vi "First Step.vi"(8 "error in (no error)":errorcluster, 11 "Wavelength PEM and Digikröm.lvclass in":refnum<class "Wavelength PEM and Digikröm.lvclass">) -> (0 "error out":errorcluster, 2 "Current Position":dbl, 3 "Wavelength PEM and Digikröm.lvclass out":refnum<class "Wavelength PEM and Digikröm.lvclass">)   [LabVIEW 2017, in "Wavelength PEM and Digikröm.lvclass"]
doc: "(Dynamic) Reset the instrument and prepare to scan. Go to step #0 - the first step. If desired, the scanner may do this in a different way than usual (i.e. by preparing to move a long distance, or reset to home position.)"
uses:
  Scanner/Scanner.lvclass
  Instruments/Utility Classes/Scannable/Scannable.lvclass
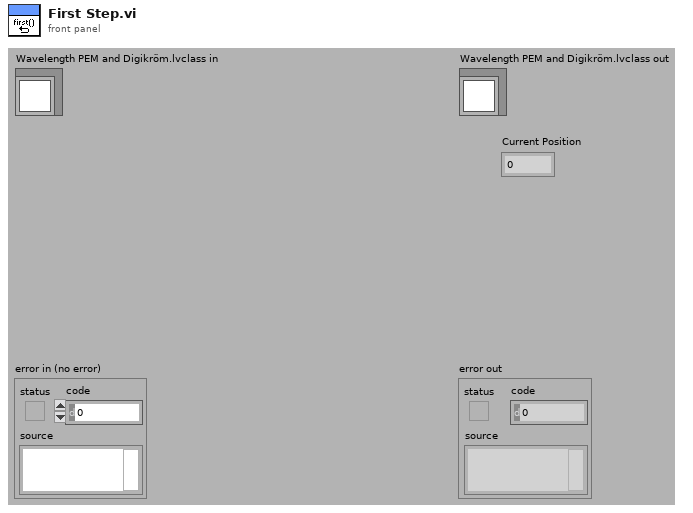
[diagram p1: front panel]
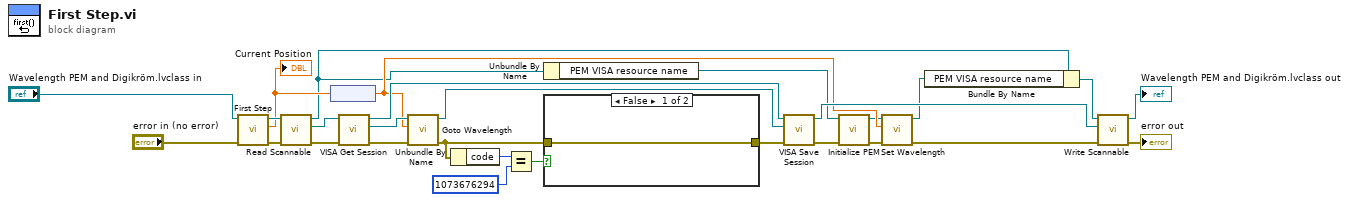
[diagram p0: block diagram]
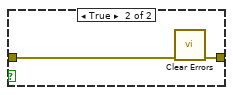
[diagram p2: hidden frame]
diagram:
  n1 = call-parent "First Step.vi"("error in (no error)"="error in (no error)", "Scanner.lvclass in"="Wavelength PEM and Digikröm.lvclass in") -> ("error out"=w20:errorcluster, "Current Position"=w13:dbl, "Scanner.lvclass out"=w24:refnum<class "Wavelength PEM and Digikröm.lvclass">)  [unwired: 7 out]
  "Current Position" <- w13
  n2 = call-dynamic "Read Scannable.vi"("error in (no error)"=w20, "Scanner.lvclass in"=w24) -> ("error out"=w19:errorcluster, "Scannable.lvclass"=w23:refnum<class "Scannable.lvclass">, "Scanner.lvclass out"=w8:refnum<class "Wavelength PEM and Digikröm.lvclass">)  [unwired: 7 out]
  n3 = node(w13) -> (w10:dbl[unit])
  n4 = call-dynamic "VISA Get Session.vi"("error in (no error)"=w19, "Instrument.lvclass in"=w23) -> ("error out"=w18:errorcluster, "VISA Resource Name"=w22:refnum<visa-resource-name>, "Instrument.lvclass out"=w16:refnum<class "Scannable.lvclass">)  [unwired: 7 out]
  n5 = call "Goto Wavelength.vi"("error in (no error)"=w18, "WAVELENGTH"=w10, "VISA resource name"=w22) -> ("error out"=w28:errorcluster, "VISA resource name out"=w21:refnum<visa-resource-name>)  [unwired: 7 out]
  n6 = Unbundle By Name(w28) -> ("code"=w26:i32)
  n7 = Equal?(x=w26, y=1073676294) -> (x = y?=w25:bool)
  n8 = Unbundle By Name(w8) -> ("PEM VISA resource name"=w1:refnum<visa-resource-name>)
  n9 = case shown="False" w25 {
    tunnel: w28 -> [w29 w31]
    tunnel: [w29 w30] -> w6
    frame False {
    }
    frame True {
      n10 = call <vilib>:"Clear Errors.vi"("error in (no error)"=w31) -> ("error out"=w30:errorcluster)  [unwired: 5 in, 1 out]
    }
  }
  n11 = call-dynamic "VISA Save Session.vi"("error in (no error)"=w6, "VISA Resource Name"=w21, "Instrument.lvclass in"=w16) -> ("error out"=w4:errorcluster, "Instrument.lvclass out"=w17:refnum<class "Scannable.lvclass">)  [unwired: 7 out]
  n12 = call "Initialize PEM.vi"("error in (no error)"=w4, "VISA resource name"=w1) -> ("error out"=w3:errorcluster, "VISA resource name out"=w2:refnum<visa-resource-name>)  [unwired: 8 in]
  n13 = call "Set Wavelength.vi"("error in (no error)"=w3, "wavelength"=w10, "VISA resource name"=w2) -> ("error out"=w5:errorcluster, "VISA resource name out"=w9:refnum<visa-resource-name>)  [unwired: 5 in, 2 out]
  n14 = Bundle By Name(cluster=w8, "PEM VISA resource name"=w9) -> (w7:refnum<class "Wavelength PEM and Digikröm.lvclass">)
  n15 = call-dynamic "Write Scannable.vi"("error in (no error)"=w5, "Scannable.lvclass"=w17, "Scanner.lvclass in"=w7) -> ("error out"=→"error out":errorcluster, "Scanner.lvclass out"=→"Wavelength PEM and Digikröm.lvclass out":refnum<class "Wavelength PEM and Digikröm.lvclass">)  [unwired: 7 out]
